vi "String To 1D DBL.vi"(7 "Delimiter":string=",", 10 "String In":string) -> (2 "1D DBL Out":dbl[](array[numeric]) format="%#_f")   [LabVIEW 2024]
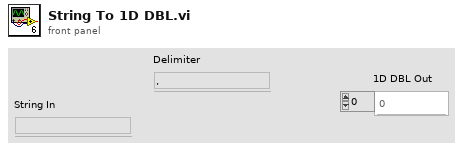
[diagram p1: front panel]
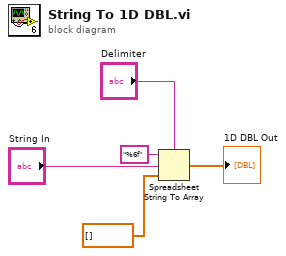
[diagram p0: block diagram]
diagram:
  n1 = Spreadsheet String To Array(delimiter (Tab)="Delimiter", format string="%6f", spreadsheet string="String In", array type (2D Dbl)=dbl[] []) -> (array=→"1D DBL Out":dbl[])
